vi "保存配置.vi"(11 "输入簇":T1) -> ()   [LabVIEW 2016, in "数据查询.lvlib"]
uses:
  <vilib>/Utility/config.llb/NI_LVConfig.lvlib
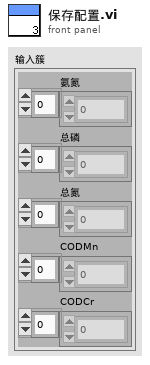
[diagram p1: front panel]
types:
  T1 = cluster{"氨氮":dbl[], "总磷":dbl[], "总氮":dbl[], "CODMn":dbl[], "CODCr":dbl[]}
  T2 = typedef "NI_LVConfig.lvlib/Config Data RefNum.ctl" = refnum<k1>
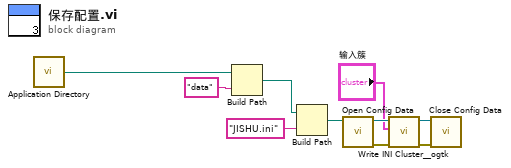
[diagram p0: block diagram]
diagram:
  n1 = call <vilib>:"Application Directory.vi"() -> ("Application Directory"=w1:path)
  n2 = Build Path(base path=w1, name or relative path="data" ("名称或相对路径")) -> (appended path=w3:path)
  n3 = Build Path(base path=w3, name or relative path="JISHU.ini" ("名称或相对路径")) -> (appended path=w5:path)
  n4 = call <vilib>:"Open Config Data.vi"("configuration file path"=w5) -> ("error out"=w8:errorcluster, "refnum"=w7:T2)  [unwired: 8 in, 1 out]
  n5 = call <userlib>:"Write INI Cluster__ogtk.vi"("error in (no error)"=w8, "INI Fomatted Cluster"="输入簇", "refnum"=w7) -> ("error out"=w9:errorcluster, "dup refnum"=w10:T2)  [unwired: 7 in]
  n6 = call <vilib>:"Close Config Data.vi"("error in (no error)"=w9, "refnum"=w10) -> ()  [unwired: 8 in, 2 out]
